vi "Post Webmessage.vi"(8 "Error In":errorcluster, 11 "object in":refnum<class "WebView.lvclass">) -> (0 "Error Out":errorcluster, 3 "object out":refnum<class "WebView.lvclass">)   [LabVIEW 2024, in "WebView.lvclass"]
uses:
  WebView.lvclass
  WebView.lvclass/WebView.ctl
  <vilib>/sklein/WebView2/Libs/Microsoft.Web.WebView2.Core.dll
panel:
  in  "Send as JSON":bool
  in  "Message":string
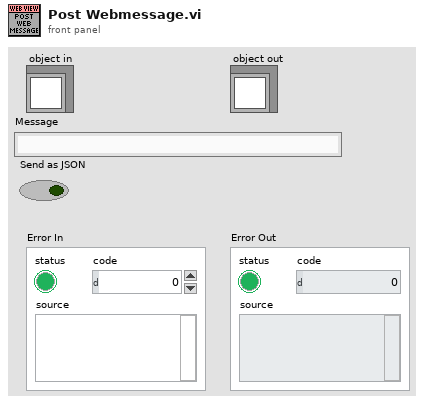
[diagram p1: front panel]
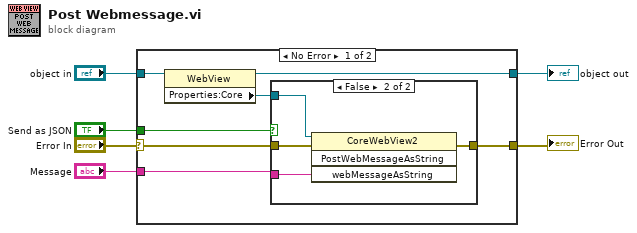
[diagram p0: block diagram]
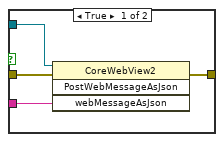
[diagram p2: hidden frame]
diagram:
  n1 = case shown="No Error" "Error In" {
    selector: "Error In" -> [w8 w23]
    tunnel: [w7 w23] -> w5
    tunnel: [w12 w22] -> w3
    tunnel: "object in" -> [w13 w22]
    tunnel: "Message" -> [w11 _]
    tunnel: "Send as JSON" -> [w10 _]
    frame No Error {
      n2 = property class="WebView"(reference=w13) -> (reference out=w12:refnum<class "WebView.lvclass">, "Properties:Core"=w9:refnum<k24>)  [unwired: 1 in, 1 out]
      n3 = case shown="False" w10 {
        tunnel: w9 -> [w17 w21]
        tunnel: w11 -> [w16 w20]
        tunnel: w8 -> [w15 w18]
        tunnel: [w14 w19] -> w7
        frame True {
          n4 = invoke class="CoreWebView2" method="PostWebMessageAsJson"(reference=w17, error in=w15, "webMessageAsJson"=w16) -> (error out=w14:errorcluster)  [unwired: 1 in, 3 out]
        }
        frame False {
          n5 = invoke class="CoreWebView2" method="PostWebMessageAsString"(reference=w21, error in=w18, "webMessageAsString"=w20) -> (error out=w19:errorcluster)  [unwired: 1 in, 3 out]
        }
      }
    }
    frame Error {
    }
  }
  "Error Out" <- w5
  "object out" <- w3
